vi "Insert Neighborhood.vi"(8 "w":i32, 9 "y":i32, 10 "Generate Random Indices?":bool, 11 "C'":u16[](array[numeric])) -> (3 "Chromosome Out":u16[](array[numeric]))   [LabVIEW 2013]
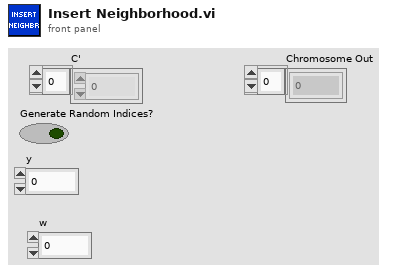
[diagram p1: front panel]
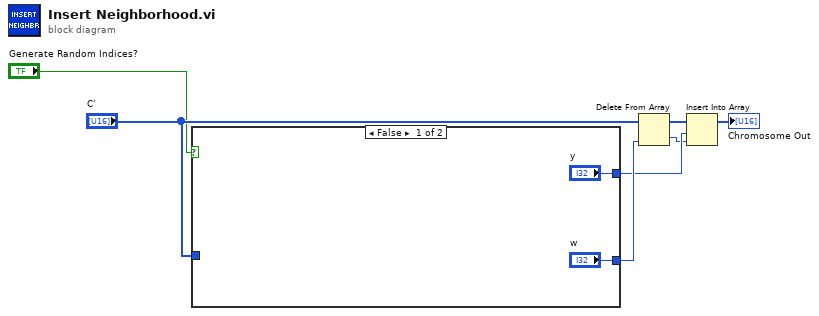
[diagram p0: block diagram]
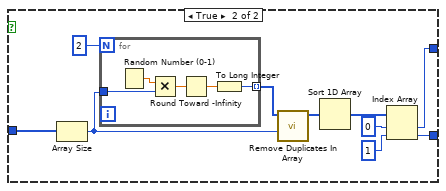
[diagram p2: hidden frame]
diagram:
  n1 = case shown="False" "Generate Random Indices?" {
    tunnel: "C'" -> [_ w19]
    tunnel: ["w" w11] -> w4
    tunnel: ["y" w10] -> w3
    frame False {
    }
    frame True {
      n2 = Array Size(array=w19) -> (size(s)=w16:i32)
      n3 = for {
        N: 2 -> [_]
        tunnel: w16 -> [w23]
        tunnel: [w20] -> w17 mode=indexing
        n4 = Random Number (0-1)() -> (number: 0 to 1=w24:dbl)
        n5 = Multiply(x=w24, y=w23) -> (x*y=w22:dbl)
        n6 = Round Toward -Infinity(1:w22) -> (0:w21:dbl)
        n7 = To Long Integer(number=w21) -> (32bit integer=w20:i32)
      }
      n8 = call "Remove Duplicates In Array.vi"("Max Index Bound"=w16, "Random Numbers Array"=w17) -> ("Random Numbers Array without Duplicates"=w13:i32[])  [unwired: 9 in]
      n9 = Sort 1D Array(array=w13) -> (sorted array=w12:i32[])
      n10 = Index Array(array=w12, index #1=0 ("index"), index #2=1 ("index")) -> (element #1=w10:i32, element #2=w11:i32)
    }
  }
  n11 = Delete From Array(array="C'", index=w4) -> (deleted portion=w2:u16, array with subset deleted=w5:u16[])  [unwired: 1 in]
  n12 = Insert Into Array(array=w5, index=w3, new element=w2) -> (→"Chromosome Out":u16[])
